vi "Main.vi"() -> ()   [LabVIEW 2022 SP3]
panel:
  out "Output":dbl
  in  "Enum":enum16{"Parallelschaltung", "Serienschaltung"}(ring)=enum."Serienschaltung"
  in  "Widerstände R":dbl[](array[numeric])
  in  "Numeric":u8
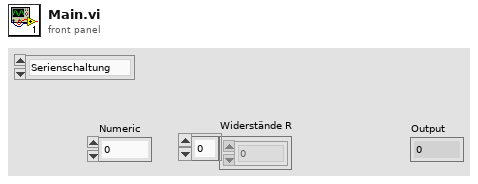
[diagram p1: front panel]
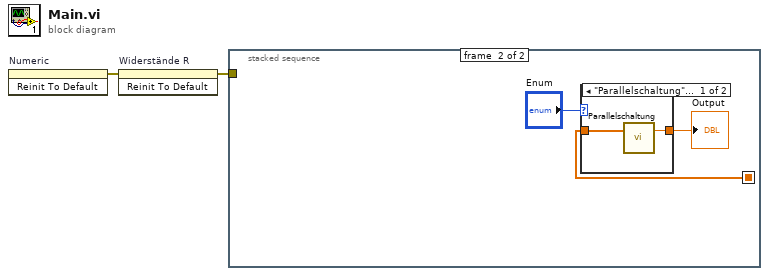
[diagram p0: block diagram]
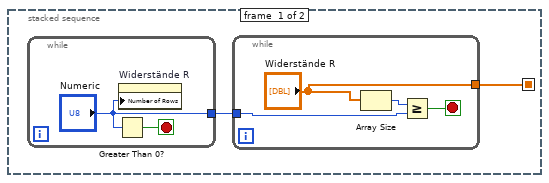
[diagram p2: hidden frame]
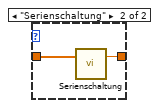
[diagram p3: hidden frame]
diagram:
  n1 = invoke on="Numeric" class="DigNum (strict)" method="Reinit To Default"() -> (error out=w2:errorcluster)  [unwired: 3 in, 2 out]
  n2 = invoke on="Widerstände R" class="Arr (strict)" method="Reinit To Default"(error in=w2) -> (error out=w1:errorcluster)  [unwired: 2 in, 2 out]
  n3 = stacked-sequence {
    seq-local: [w3 _] -> [_ w12]
    tunnel: w1 -> [_ _]
    frame #0 {
      n4 = while {
        tunnel: ["Numeric"] -> w4
        stop <- w10 stop-if-true
        n5 = Greater Than 0?(x="Numeric") -> (x > 0?=w10:bool)
        n6 = property on="Widerstände R" class="Arr (strict)"("Number of Rows"="Numeric") -> ()  [unwired: 2 in, 2 out]
      }
      n7 = while {
        tunnel: w4 -> [w6]
        tunnel: ["Widerstände R"] -> w3
        stop <- w8 stop-if-true
        n8 = Array Size(array="Widerstände R") -> (size(s)=w7:i32)
        n9 = Greater Or Equal?(x=w7, y=w6) -> (x >= y?=w8:bool)
      }
    }
    frame #1 {
      n10 = case shown="\"Parallelschaltung\", Default" "Enum" {
        tunnel: w12 -> [w15 w17]
        tunnel: [w14 w16] -> w11
        frame "Parallelschaltung", Default {
          # "Parallel"
          n11 = call "Parallelschaltung.vi"("Array In"=w15) -> ("Out"=w14:dbl)  [unwired: 1 in, 1 out]
        }
        frame "Serienschaltung" {
          # "Seriell"
          n12 = call "Serienschaltung.vi"("Array In"=w17) -> ("Out"=w16:dbl)  [unwired: 1 in, 1 out]
        }
      }
      "Output" <- w11
    }
  }
